vi "Configure-temperature-display.vi"(8 "error in":errorcluster, 10 "Data ref. in":refnum<data-value>, 11 "UI ref. in":refnum<data-value>) -> (0 "error IO":errorcluster, 2 "Data ref.":refnum<data-value>, 3 "UI ref.":refnum<data-value>)   [LabVIEW 2013, in "CameraVision.lvlib" / "CV-UI.lvclass"]
doc: "This function calculates the values for the x-and y-axes of the temperature graph.\nThe scale is based on the parameters from the 'Configuration' tab, while the center of the graph is determined by the 'Axis origin relative position' hidden parameter (0 = top-left of image, 0.5 = center of image, 1 = bottom right of image)."
uses:
  CV-UI.lvclass
  Main/CV-Main.lvclass
  Display-names.ctl
  CV-UI.lvclass/CV-UI.ctl
  Main/CV-Main.lvclass/CV-Main.ctl
  Read Display refs.vi
  Main/Read Temperature params.vi
  Main/Read Config params.vi
  Main/Temperature/CV-Temperature.lvclass
  Main/Configuration/CV-Configuration.lvclass
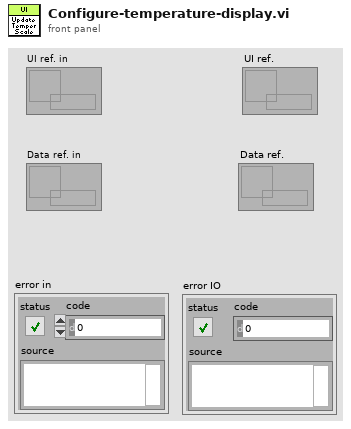
[diagram p1: front panel]
types:
  T1 = typedef "CameraVision.lvlib/CV-UI.lvclass/Display-names.ctl" = enum16{"State", "Action", "Current image", "Framerate", "Frametime", "Process buffer", "Storage buffer", "Free disk space", "Total disk space", "Information", "Histogram", "Camera 1", "Camera 2", "Camera 1 chart", "Camera 2 chart", "Browser", "Temperature", "Map", "Status overview", "Characteristics", "Temper characteristics"}
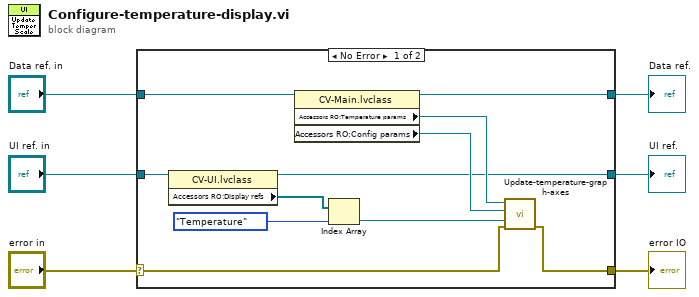
[diagram p0: block diagram]
diagram:
  n1 = case shown="No Error" "error in" {
    selector: "error in" -> [w13 w20]
    tunnel: [w17 w20] -> w6
    tunnel: "Data ref. in" -> [w11 w18]
    tunnel: "UI ref. in" -> [w14 w19]
    tunnel: [w10 w18] -> w2
    tunnel: [w12 w19] -> w1
    frame No Error {
      n2 = property class="CV-UI.lvclass"(reference=w14) -> (reference out=w12:refnum<data-value>, "Accessors RO:Display refs"=w9:refnum<vi>[])  [unwired: 1 in, 1 out]
      n3 = property class="CV-Main.lvclass"(reference=w11) -> (reference out=w10:refnum<data-value>, "Accessors RO:Temperature params"=w16:refnum<data-value>, "Accessors RO:Config params"=w15:refnum<data-value>)  [unwired: 1 in, 1 out]
      n4 = Index Array(array=w9, index=Display-names."Temperature" ("Dislay")) -> (element=w7:refnum<vi>)
      n5 = call "Update-temperature-graph-axes.vi"("error in (no error)"=w13, "Temperature graph"=w7, "Config params in"=w15, "Temperature params in"=w16) -> ("error out"=w17:errorcluster)  [unwired: 7 in]
    }
    frame Error {
    }
  }
  "error IO" <- w6
  "UI ref." <- w1
  "Data ref." <- w2
